vi "Miernik(HP-dvm1).vi"(8 "error in (no error)":errorcluster, 10 "write buffer":string, 11 "VISA Refnum in":refnum<visa-resource-name>) -> (0 "error out":errorcluster, 2 "read buffer":string, 3 "VISA Refnum out":refnum<visa-resource-name>)   [LabVIEW 2020]
uses:
  lib/VirtualLab.lvlibp/VISASimulator/VISALib.lvlib
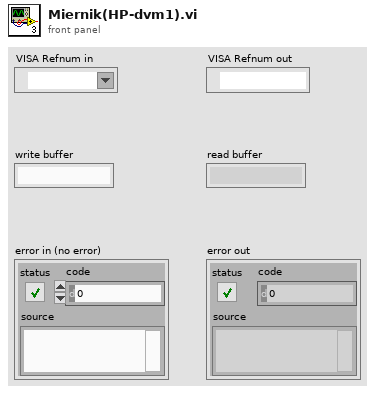
[diagram p1: front panel]
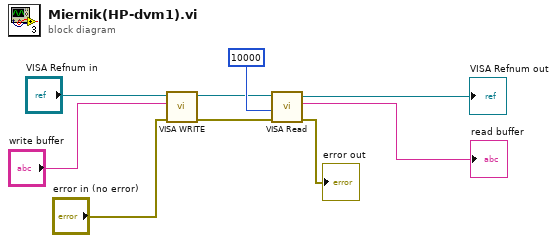
[diagram p0: block diagram]
diagram:
  n1 = call "VISA WRITE.vi"("error in (no error)"="error in (no error)", "write buffer"="write buffer", "VISA resource name"="VISA Refnum in") -> ("error out"=w7:errorcluster, "VISA resource name out"=w2:refnum<visa-resource-name>)  [unwired: 6 in, 1 out]
  n2 = call "VISA Read.vi"("error in (no error)"=w7, "byte count"=u32 10000, "VISA resource name"=w2) -> ("error out"=→"error out":errorcluster, "read buffer"=→"read buffer":string, "VISA resource name out"=→"VISA Refnum out":refnum<visa-resource-name>)  [unwired: 5 in, 1 out]
